vi "KeithleyMonitor.vi"   [LabVIEW 2019]
uses:
  Instrument_Setup.vi
  Global/Global Variables/Data_Display_global.vi
  Equipment/Keithley 24XX/Public/Data/Read (Single Point).vi
  Equipment/Keithley 24XX/Keithley 24XX.lvlib
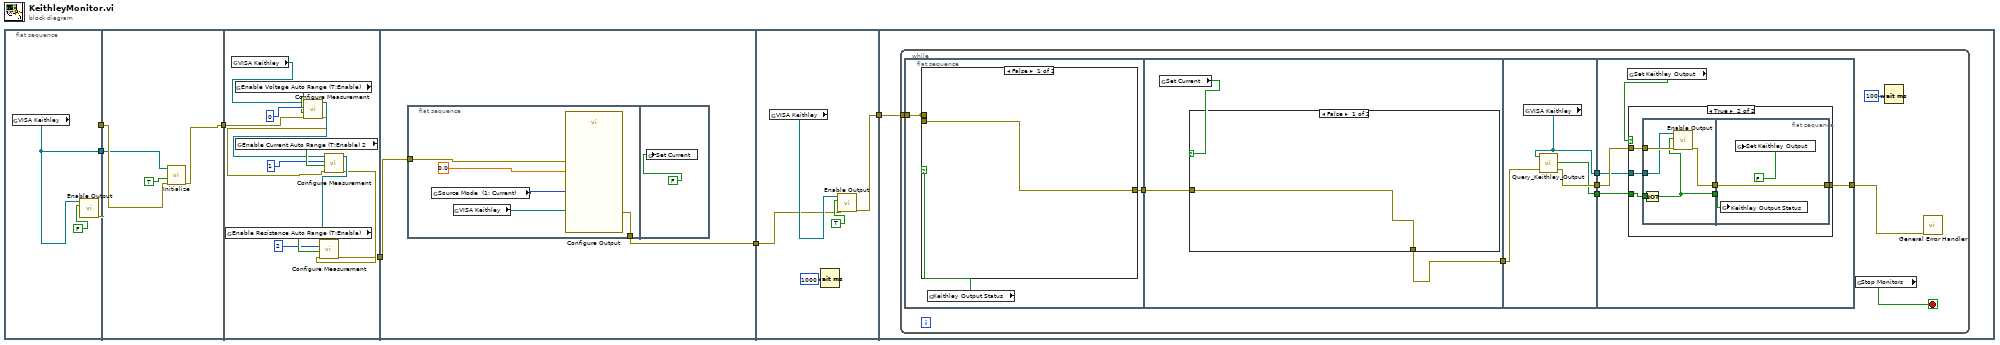
[diagram p0: block diagram]
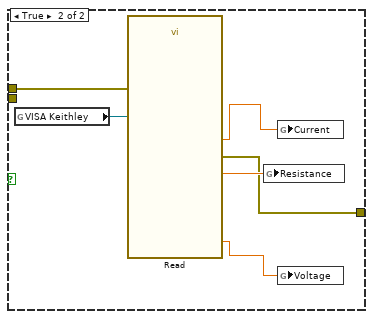
[diagram p2: hidden frame]
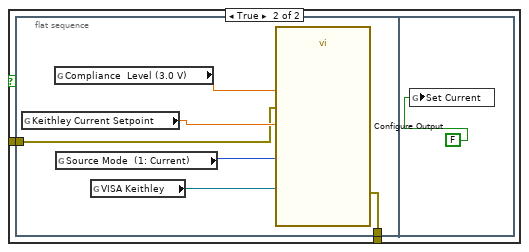
[diagram p3: hidden frame]
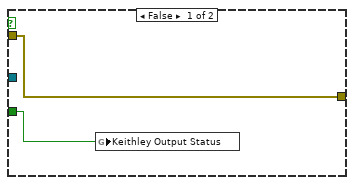
[diagram p4: hidden frame]
diagram:
  n1 = flat-sequence {
    tunnel: [w8] -> w4
    tunnel: [w7] -> w2
    tunnel: w4 -> [w12]
    tunnel: [w11] -> w3
    tunnel: w2 -> [w10]
    tunnel: [w15] -> w6
    tunnel: w3 -> [w14]
    tunnel: w6 -> [w28]
    tunnel: [w27] -> w5
    tunnel: w5 -> [w36]
    tunnel: [w35] -> w1
    tunnel: w1 -> [w40]
    frame #0 {
      n2 = global read "Instrument_Setup.vi" "VISA Keithley"() -> (w7:refnum<visa-resource-name>)
      n3 = call "Enable Output.vi"("Enable Output (T: Enable)"=FALSE, "VISA resource name"=w7) -> ("error out"=w8:errorcluster)  [unwired: 8 in, 1 out]
    }
    frame #1 {
      n4 = call "Initialize.vi"("error in (no error)"=w12, "Reset (True)"=TRUE, "VISA resource name"=w10) -> ("error out"=w11:errorcluster)  [unwired: 7 in, 1 out]
    }
    frame #2 {
      n5 = global read "Instrument_Setup.vi" "Enable Resistance Auto Range (T:Enable)"() -> (w26:bool)
      n6 = global read "Instrument_Setup.vi" "VISA Keithley"() -> (w20:refnum<visa-resource-name>)
      n7 = global read "Instrument_Setup.vi" "Enable Voltage Auto Range (T:Enable)"() -> (w21:bool)
      n8 = global read "Instrument_Setup.vi" "Enable Current Auto Range (T:Enable) 2"() -> (w25:bool)
      n9 = call "Configure Measurement.vi"("error in (no error)"=w14, "Enable Auto Range (T:Enable)"=w21, "Function (0: Volts)"=0, "VISA resource name"=w20) -> ("error out"=w17:errorcluster, "VISA resource name out"=w19:refnum<visa-resource-name>)  [unwired: 6 in]
      n10 = call "Configure Measurement.vi"("error in (no error)"=w17, "Enable Auto Range (T:Enable)"=w25, "Function (0: Volts)"=1, "VISA resource name"=w19) -> ("error out"=w16:errorcluster, "VISA resource name out"=w18:refnum<visa-resource-name>)  [unwired: 6 in]
      n11 = call "Configure Measurement.vi"("error in (no error)"=w16, "Enable Auto Range (T:Enable)"=w26, "Function (0: Volts)"=2, "VISA resource name"=w18) -> ("error out"=w15:errorcluster)  [unwired: 6 in, 1 out]
    }
    frame #3 {
      n12 = flat-sequence {
        tunnel: w28 -> [w30]
        tunnel: [w29] -> w27
        frame #0 {
          n13 = global read "Instrument_Setup.vi" "Source Mode  (1: Current)"() -> (w32:u16)
          n14 = global read "Instrument_Setup.vi" "VISA Keithley"() -> (w33:refnum<visa-resource-name>)
          n15 = call "Configure Output.vi"("Source Mode  (0: Voltage)"=w32, "error in (no error)"=w30, "Output Level (0)"=0.0, "VISA resource name"=w33) -> ("error out"=w29:errorcluster)  [unwired: 6 in, 1 out]
        }
        frame #1 {
          n16 = global write "Data_Display_global.vi" "Set Current"(FALSE) -> ()
        }
      }
    }
    frame #4 {
      n17 = global read "Instrument_Setup.vi" "VISA Keithley"() -> (w39:refnum<visa-resource-name>)
      n18 = Wait (ms)(milliseconds to wait=1000) -> ()  [unwired: 1 out]
      n19 = call "Enable Output.vi"("error in (no error)"=w36, "Enable Output (T: Enable)"=TRUE, "VISA resource name"=w39) -> ("error out"=w35:errorcluster)  [unwired: 7 in, 1 out]
    }
    frame #5 {
      n20 = while {
        tunnel: w40 -> [w47]
        stop <- w49 stop-if-true
        n21 = flat-sequence {
          tunnel: w47 -> [w50]
          tunnel: [w52] -> w46
          tunnel: w46 -> [w61]
          tunnel: [w60] -> w45
          tunnel: w45 -> [w76]
          tunnel: [w75] -> w43
          tunnel: [w74] -> w42
          tunnel: [w73] -> w41
          tunnel: [w79] -> w44
          tunnel: w43 -> [w80]
          tunnel: w42 -> [w78]
          tunnel: w41 -> [w77]
          frame #0 {
            n22 = global read "Data_Display_global.vi" "Keithley Output Status"() -> (w51:bool)
            n23 = case shown="False" w51 {
              tunnel: w50 -> [_ w55]
              tunnel: [w53 w54] -> w52
              tunnel: w50 -> [w53 _]
              frame False {
              }
              frame True {
                n24 = global read "Instrument_Setup.vi" "VISA Keithley"() -> (w59:refnum<visa-resource-name>)
                n25 = call-poly "Read.vi"("VISA resource name"=w59, "error in (no error)"=w55) -> ("Voltage"=w57:sgl, "Current"=w58:sgl, "Resistance"=w56:sgl, "error out"=w54:errorcluster)  [unwired: 7 in, 3 out]
                n26 = global write "Data_Display_global.vi" "Resistance"(w56) -> ()
                n27 = global write "Data_Display_global.vi" "Current"(w58) -> ()
                n28 = global write "Data_Display_global.vi" "Voltage"(w57) -> ()
              }
            }
          }
          frame #1 {
            n29 = global read "Data_Display_global.vi" "Set Current"() -> (w62:bool)
            n30 = case shown="False" w62 {
              tunnel: w61 -> [w63 w65]
              tunnel: [w63 w64] -> w60
              frame False {
              }
              frame True {
                n31 = flat-sequence {
                  tunnel: w65 -> [w67]
                  tunnel: [w66] -> w64
                  frame #0 {
                    n32 = global read "Data_Display_global.vi" "Keithley Current Setpoint"() -> (w68:dbl)
                    n33 = global read "Instrument_Setup.vi" "Compliance  Level (3.0 V)"() -> (w70:dbl)
                    n34 = global read "Instrument_Setup.vi" "Source Mode  (1: Current)"() -> (w69:u16)
                    n35 = global read "Instrument_Setup.vi" "VISA Keithley"() -> (w71:refnum<visa-resource-name>)
                    n36 = call "Configure Output.vi"("Source Mode  (0: Voltage)"=w69, "error in (no error)"=w67, "Compliance  Level (3.0V)"=w70, "Output Level (0)"=w68, "VISA resource name"=w71) -> ("error out"=w66:errorcluster)  [unwired: 5 in, 1 out]
                  }
                  frame #1 {
                    n37 = global write "Data_Display_global.vi" "Set Current"(FALSE) -> ()
                  }
                }
              }
            }
          }
          frame #2 {
            n38 = global read "Instrument_Setup.vi" "VISA Keithley"() -> (w74:refnum<visa-resource-name>)
            n39 = call "Query_Keithley_Output.vi"("error in (no error)"=w76, "VISA resource name"=w74) -> ("error out"=w75:errorcluster, "Output"=w73:bool)  [unwired: 1 in, 1 out]
          }
          frame #3 {
            n40 = global read "Data_Display_global.vi" "Set Keithley Output"() -> (w81:bool)
            n41 = case shown="True" w81 {
              tunnel: w80 -> [w83 w89]
              tunnel: [w83 w88] -> w79
              tunnel: w78 -> [_ w87]
              tunnel: w77 -> [w82 w86]
              frame False {
                n42 = global write "Data_Display_global.vi" "Keithley Output Status"(w82) -> ()
              }
              frame True {
                n43 = flat-sequence {
                  tunnel: w89 -> [w94]
                  tunnel: w87 -> [w92]
                  tunnel: w86 -> [w91]
                  tunnel: [w93] -> w85
                  tunnel: [w90] -> w84
                  tunnel: [w97] -> w88
                  tunnel: w85 -> [w97]
                  tunnel: w84 -> [w95]
                  frame #0 {
                    n44 = Not(x=w91) -> (.not. x?=w90:bool)
                    n45 = call "Enable Output.vi"("error in (no error)"=w94, "Enable Output (T: Enable)"=w90, "VISA resource name"=w92) -> ("error out"=w93:errorcluster)  [unwired: 7 in, 1 out]
                  }
                  frame #1 {
                    n46 = global write "Data_Display_global.vi" "Keithley Output Status"(w95) -> ()
                    n47 = global write "Data_Display_global.vi" "Set Keithley Output"(FALSE) -> ()
                  }
                }
              }
            }
          }
        }
        n48 = global read "Data_Display_global.vi" "Stop Monitors"() -> (w49:bool)
        n49 = Wait (ms)(milliseconds to wait=100) -> ()  [unwired: 1 out]
        n50 = call <vilib>:"General Error Handler.vi"("error in (no error)"=w44) -> ()  [unwired: 10 in, 5 out]
      }
    }
  }
